vi "TrackerTTLsignal_171213.vi"(11 "Serial Port":refnum<visa-resource-name>) -> ()   [LabVIEW 2016]
doc: "This example demonstrates how to write N channels of digital ouput from a LINX device."
uses:
  Globaltracker.vi
panel:
  in  "Tab Control":enum32{"Page 1", "Page 2"}(tab)
  out "Total number":string
  out "seconds":string
  out "TTL is on":string
  out "ON/OFF":bool
  out "TotalNumberOf Events":dbl
  out "TTLduration":u32
  out "LED control setting:":string
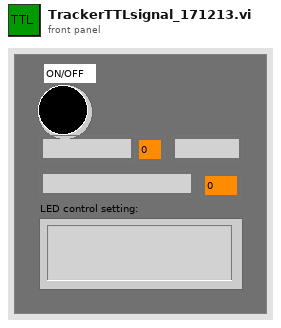
[diagram p1: front panel]
types:
  T1 = cluster{"Region number":i32, "ON/OFF":bool, "Activation type":string, "Activation critaria":i32, "Reward":i32}[]
  T2 = cluster{"Region number":i32, "ON/OFF":bool, "Activation type":string, "Activation critaria":i32, "Reward":i32}
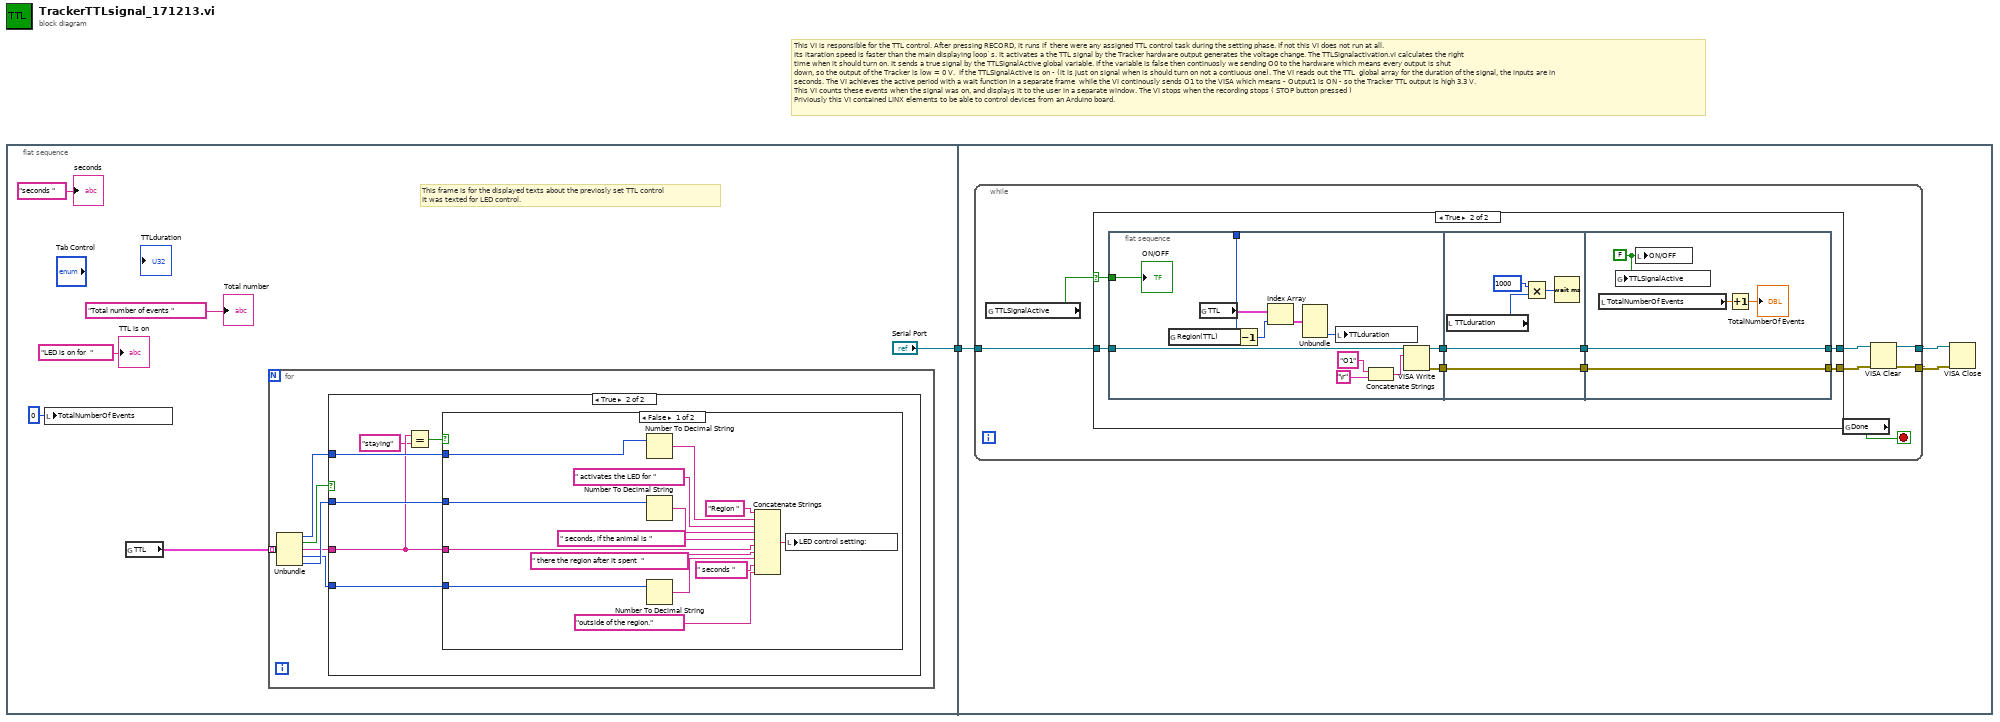
[diagram p0: block diagram]
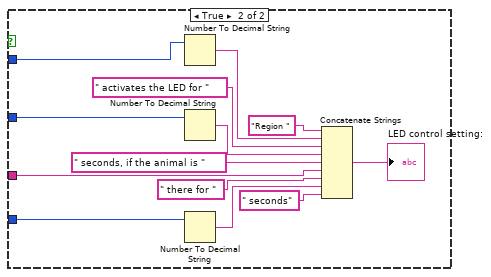
[diagram p3: hidden frame]
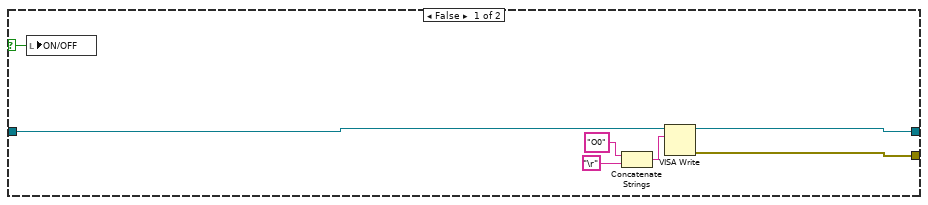
[diagram p4: hidden frame]
diagram:
  # "This VI is responsible for the TTL control. After pressing RECORD, it runs if  there were any assigned TTL control task during the setting phase. If not this VI does not run at all.\nIts itaration speed is faster than the main displaying loop`s. It activates a the TTL signal by the Tracker hardware output generates the voltage change. The TTLSignalactivation.vi calculates the right\ntime when it should turn on. It sends a true signal by the TTLSignalActive global variable. If the variable is false then continuosly we sending O0 to the hardware which means every output is shut\ndown, so the output of the Tracker is low = 0 V.  If the TTLSignalActive is on - (it is just on signal when is should turn on not a contiuous one). The VI reads out the TTL  global array for the duration of the signal, the inputs are in seconds. The VI achieves the active period with a wait function in a separate frame  while the VI continously sends O1 to the VISA which means - Output1 is ON - so the Tracker TTL output is high 3.3 V.\nThis VI counts these events when the signal was on, and displays it to the user in a separate window. The VI stops when the recording stops ( STOP button pressed )\nPriviously this VI contained LINX elements to be able to control devices from an Arduino board."
  n1 = flat-sequence {
    tunnel: ["Serial Port"] -> w1
    tunnel: w1 -> [w49]
    frame #0 {
      # "This frame is for the displayed texts about the previosly set TTL control \nIt was texted for LED control."
      n2 = local write "TotalNumberOf Events"(u8 0 ("NumberOfRewardWasGiven")) -> ()
      n3 = global read "Globaltracker.vi" "TTL"() -> (w2:T1)
      n4 = for {
        tunnel: w2 -> [w13] mode=indexing
        n5 = Unbundle(w13) -> ("Region number"=w11:i32, "ON/OFF"=w12:bool, "Activation type"=w9:string, "Activation critaria"=w8:i32, "Reward"=w10:i32)
        n6 = case shown="True" w12 {
          tunnel: w11 -> [_ w19]
          tunnel: w10 -> [_ w18]
          tunnel: w9 -> [_ w15]
          tunnel: w8 -> [_ w17]
          frame False {
          }
          frame True {
            n7 = Equal?(x=w15, y="staying") -> (x = y?=w16:bool)
            n8 = case shown="False" w16 {
              tunnel: w19 -> [w25 w45]
              tunnel: w18 -> [w24 w42]
              tunnel: w15 -> [w22 w39]
              tunnel: w17 -> [w23 w37]
              frame False {
                n9 = Number To Decimal String(number=w25) -> (decimal integer string=w32:string)  [unwired: 1 in]
                n10 = Number To Decimal String(number=w24) -> (decimal integer string=w30:string)  [unwired: 1 in]
                n11 = Number To Decimal String(number=w23) -> (decimal integer string=w27:string)  [unwired: 1 in]
                n12 = Concatenate Strings("Region ", w32, " activates the LED for " ("string"), w30, " seconds, if the animal is " ("string"), w22, " there the region after it spent  " ("string"), w27, " seconds " ("string"), "outside of the region." ("string")) -> (w20:string)
                n13 = local write "LED control setting:"(w20) -> ()
              }
              frame True {
                n14 = Number To Decimal String(number=w45) -> (decimal integer string=w44:string)  [unwired: 1 in]
                n15 = Number To Decimal String(number=w42) -> (decimal integer string=w41:string)  [unwired: 1 in]
                n16 = Number To Decimal String(number=w37) -> (decimal integer string=w36:string)  [unwired: 1 in]
                n17 = Concatenate Strings("Region ", w44, " activates the LED for " ("string"), w41, " seconds, if the animal is " ("string"), w39, " there for " ("string"), w36, " seconds" ("string")) -> (→"LED control setting:":string)
              }
            }
          }
        }
      }
      "TTL is on" <- "LED is on for  " ("String 2")
      "seconds" <- "seconds " ("String 3")
      "Total number" <- "Total number of events " ("String 4")
    }
    frame #1 {
      n18 = while {
        tunnel: w49 -> [w54]
        tunnel: [w52] -> w47
        tunnel: [w50] -> w48
        stop <- w56 stop-if-true
        n19 = global read "Globaltracker.vi" "TTLSignalActive"() -> (w55:bool)
        n20 = case shown="True" w55 {
          selector: w55 -> [w63 w71]
          tunnel: w54 -> [w62 w70]
          tunnel: [w58 w69] -> w53
          tunnel: [w57 w66] -> w51
          frame False {
            n21 = local write "ON/OFF"(w63) -> ()
            n22 = Concatenate Strings("O0" ("write buffer"), "\r") -> (w61:string)
            n23 = VISA Write(VISA resource name=w62, write buffer=w61) -> (VISA resource name out=w58:refnum<visa-resource-name>, error out=w57:errorcluster)  [unwired: 1 in, 1 out]
          }
          frame True {
            n24 = flat-sequence {
              tunnel: w71 -> [w79]
              tunnel: [w78] -> _
              tunnel: w70 -> [w74]
              tunnel: [w73] -> w67
              tunnel: [w72] -> w64
              tunnel: [w85] -> w68
              tunnel: w67 -> [w85]
              tunnel: [w84] -> w65
              tunnel: w64 -> [w84]
              tunnel: [w91] -> w69
              tunnel: w68 -> [w91]
              tunnel: [w90] -> w66
              tunnel: w65 -> [w90]
              frame #0 {
                n25 = global read "Globaltracker.vi" "Region(TTL)"() -> (w78:i32)
                n26 = global read "Globaltracker.vi" "TTL"() -> (w83:T1)
                n27 = Decrement(x=w78) -> (x-1=w80:i32)
                n28 = Index Array(array=w83, index=w80) -> (element=w82:T2)
                n29 = Unbundle(w82) -> ("Reward"=w81:i32)  [unwired: 4 out]
                n30 = local write "TTLduration"(w81) -> ()
                n31 = Concatenate Strings("O1" ("write buffer"), "\r") -> (w77:string)
                n32 = VISA Write(VISA resource name=w74, write buffer=w77) -> (VISA resource name out=w73:refnum<visa-resource-name>, error out=w72:errorcluster)  [unwired: 1 in, 1 out]
                "ON/OFF" <- w79
              }
              frame #1 {
                n33 = local read "TTLduration"() -> (w88:u32)
                n34 = Multiply(x=u32 1000, y=w88) -> (x*y=w86:u32)
                n35 = Wait (ms)(milliseconds to wait=w86) -> ()  [unwired: 1 out]
              }
              frame #2 {
                w92 = FALSE ("ON/OFF")
                n36 = local read "TotalNumberOf Events"() -> (w93:dbl)
                n37 = global write "Globaltracker.vi" "TTLSignalActive"(w92) -> ()
                n38 = local write "ON/OFF"(w92) -> ()
                n39 = Increment(x=w93) -> (x+1=→"TotalNumberOf Events":dbl)
              }
            }
          }
        }
        n40 = global read "Globaltracker.vi" "Done"() -> (w56:bool)
        n41 = VISA Clear(VISA resource name=w53, error in (no error)=w51) -> (VISA resource name out=w52:refnum<visa-resource-name>, error out=w50:errorcluster)
      }
      n42 = VISA Close(VISA resource name=w47, error in (no error)=w48) -> ()  [unwired: 1 out]
    }
  }
